vi "piezo voltage check.vi"(11 "piezo array in":dbl[](array[numeric])) -> (3 "piezo array out":dbl[](array[numeric]))   [LabVIEW 2017]
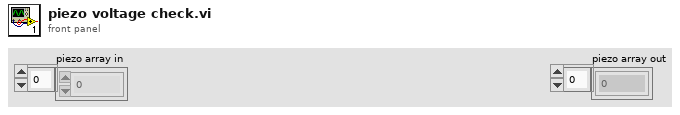
[diagram p1: front panel]
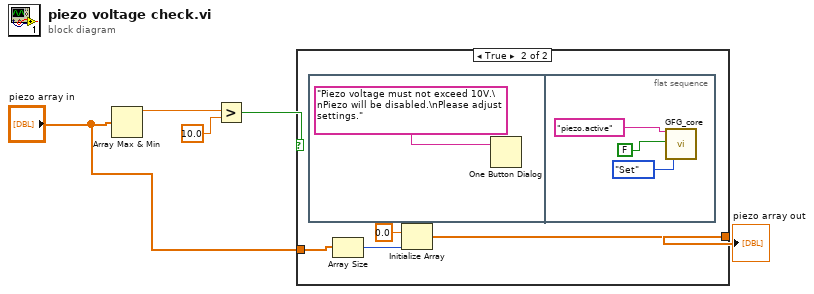
[diagram p0: block diagram]
diagram:
  n1 = Array Max & Min(array="piezo array in") -> (max value=w5:dbl)  [unwired: 3 out]
  n2 = Greater?(x=w5, y=10.0) -> (0:w3:bool)
  n3 = case shown="True" w3 {
    tunnel: "piezo array in" -> [w6 w10]
    tunnel: [w6 w7] -> w1
    frame False {
    }
    frame True {
      n4 = flat-sequence {
        frame #0 {
          n5 = One Button Dialog(message="Piezo voltage must not exceed 10V.\nPiezo will be disabled.\nPlease adjust settings.") -> ()  [unwired: 1 in, 1 out]
        }
        frame #1 {
          n6 = call "GFG_core.vi"("Variable Name in"="piezo.active", "Variant in"=FALSE ("x > y?"), "Action"=enum16{"Init", "Set", "Get", "Clear"}."Set") -> ()  [unwired: 10 in, 7 out]
        }
      }
      n7 = Array Size(array=w10) -> (size(s)=w9:i32)
      n8 = Initialize Array(0.0 ("element"), w9) -> (w7:dbl[])
    }
  }
  "piezo array out" <- w1
